vi "string test.vi"() -> ()   [LabVIEW 2021, in "Test VIs.lvclass"]
uses:
  Test VIs.lvclass
panel:
  out "number 3":u32
  out "number 2":i32
  in  "x":string
  out "x > y?":bool
  out "decimal integer string":string
  in  "width (-)":i16
  in  "number":i32
  out "number of replacements":i32
  out "offset of match":i32
  in  "string 2":string
  out "Array":string[](array[string])
  out "substring":string
  in  "length (rest)":i32
  in  "offset (0)":i32
  in  "string":string
  out "Tray":string
  in  "Tray Number":i32
  out "Position":string
  in  "Position 2":i32
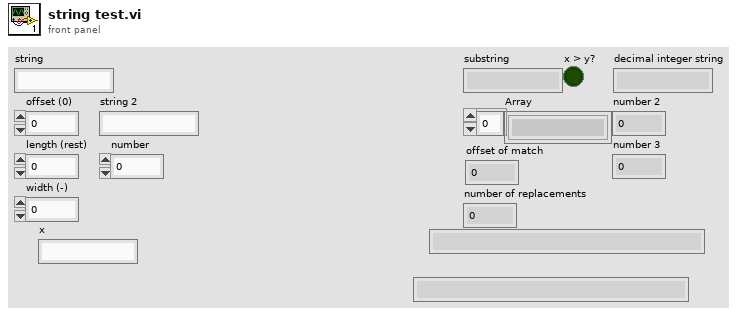
[diagram p1: front panel]
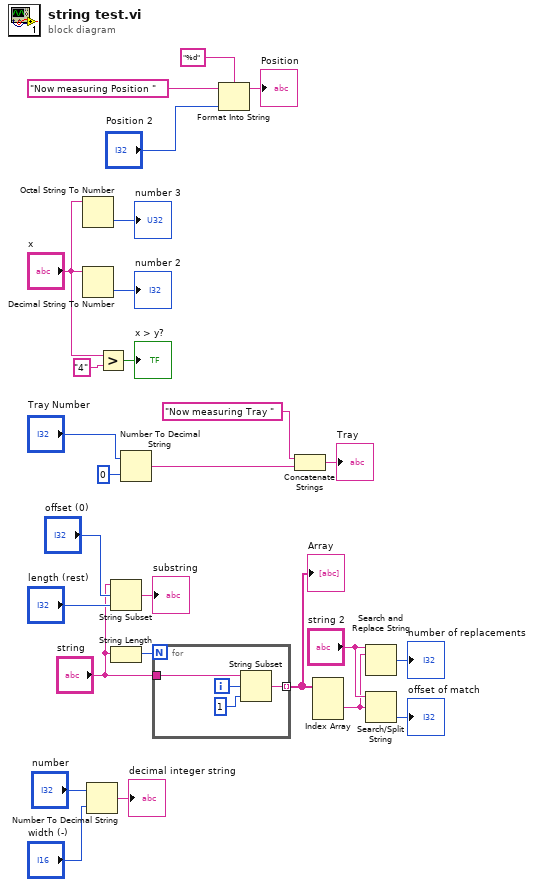
[diagram p0: block diagram]
diagram:
  n1 = Octal String To Number(4:"x") -> (0:→"number 3":u32)  [unwired: 2 in, 1 out]
  n2 = Decimal String To Number(string="x") -> (number=→"number 2":i32)  [unwired: 2 in, 1 out]
  n3 = Number To Decimal String(number="number", width (-)="width (-)") -> (decimal integer string=→"decimal integer string":string)
  n4 = Greater?(x="x", y="4") -> (0:→"x > y?":bool)
  n5 = String Subset(string="string", offset (0)="offset (0)", length (rest)="length (rest)") -> (substring=→"substring":string)
  n6 = String Length(string="string") -> (length=w15:i32)
  n7 = Number To Decimal String(number="Tray Number", width (-)=i16 0) -> (decimal integer string=w20:string)
  n8 = for {
    N: w15 -> [_]
    tunnel: [w29] -> w13 mode=indexing
    tunnel: "string" -> [w28]
    i -> [w30]
    n9 = String Subset(string=w28, offset (0)=w30, length (rest)=1 ("length (rest)")) -> (substring=w29:string)
  }
  "Array" <- w13
  n10 = Format Into String(format string="%d", initial string="Now measuring Position ", "Position 2") -> (resulting string=→"Position":string)  [unwired: 1 in, 1 out]
  n11 = Concatenate Strings("Now measuring Tray " ("string"), w20) -> (→"Tray":string)
  n12 = Index Array(array=w13) -> (element #2=w10:string)  [unwired: 3 in, 2 out]
  n13 = Search and Replace String(input string="string 2", search string=w10) -> (number of replacements=→"number of replacements":i32)  [unwired: 6 in, 3 out]
  n14 = Search/Split String(string="string 2", search string/char (-)=w10) -> (offset of match=→"offset of match":i32)  [unwired: 1 in, 2 out]
